vi "3D Axis Box Plot.vi"() -> ()   [LabVIEW 2022 SP3]
uses:
  <vilib>/Utility/miscctls.llb/LV3DPointTypeDef.ctl
  <vilib>/picture/3D Picture Control/Object/Create Object (drawable).vi
  <vilib>/picture/3D Picture Control/Object/Add Object (no reference).vi
  <vilib>/picture/3D Picture Control/NI_3D Picture Control.lvlib
panel:
  in  "Target":T1
  in  "Up Direction":T1
  in  "Camera Position":T1
  in  "Color 2":u32(colorbox)
  in  "Color":u32(colorbox)
  in  "Axis label?":bool
  in  "Half plane?":bool=TRUE
  in  "stop":bool
  out "3D Picture":refnum<vi>(3d-picture)
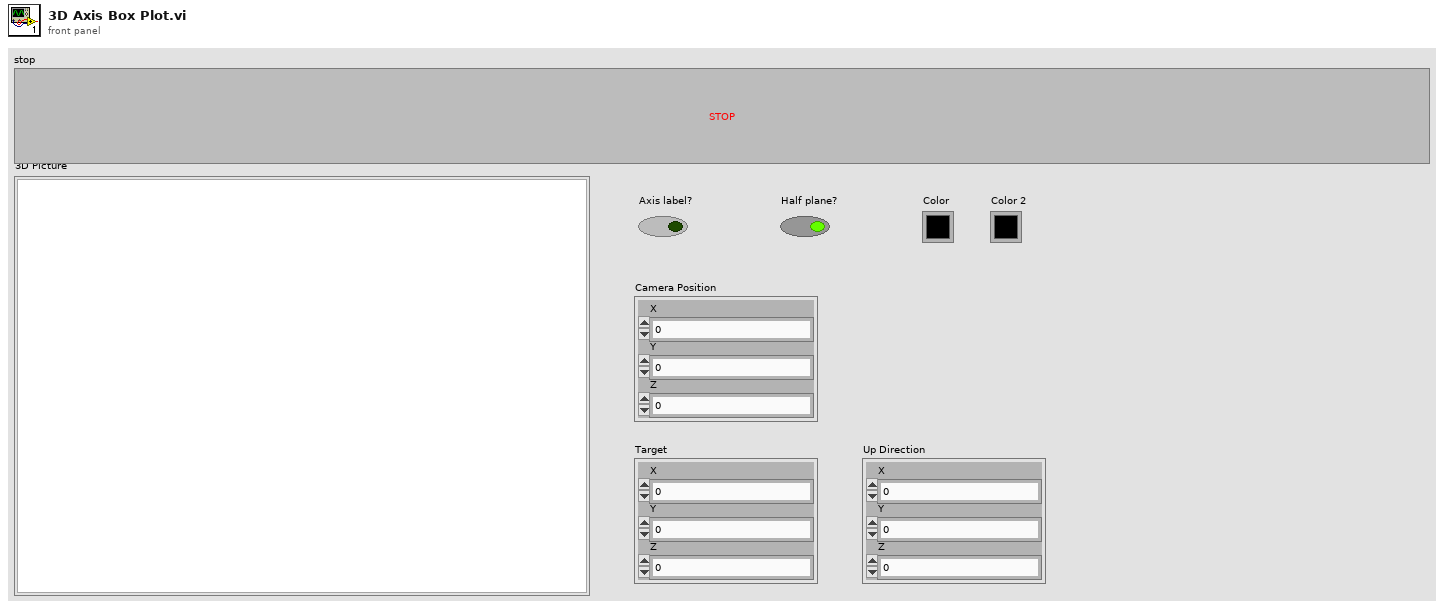
[diagram p1: front panel]
types:
  T1 = typedef "LV3DPointTypeDef.ctl" = cluster{"X":sgl, "Y":sgl, "Z":sgl}
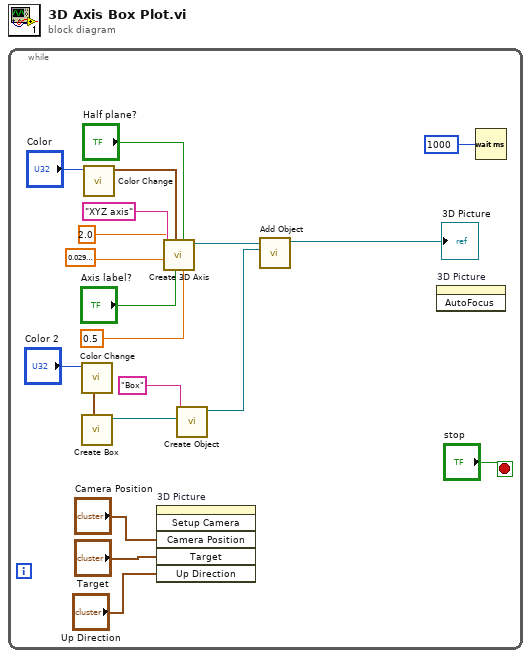
[diagram p0: block diagram]
diagram:
  n1 = while {
    stop <- "stop" stop-if-true
    n2 = call <vilib>:"Color Change.vi"("Color"="Color 2") -> ("RGBA"=w6:cluster{"R":sgl, "G":sgl, "B":sgl, "A":sgl})  [unwired: 10 in]
    n3 = call <vilib>:"Create Box.vi"("Color"=w6) -> ("New Box Refnum"=w18:refnum<vi>)  [unwired: 9 in, 1 out]
    n4 = call <vilib>:"Color Change.vi"("Color"="Color") -> ("RGBA"=w7:cluster{"R":sgl, "G":sgl, "B":sgl, "A":sgl})  [unwired: 10 in]
    n5 = invoke on="3D Picture" class="SceneGraphDisp (strict)" method="Setup Camera"("Camera Position"="Camera Position", "Target"="Target", "Up Direction"="Up Direction") -> ()  [unwired: 3 in, 6 out]
    n6 = call <vilib>:"Create 3D Axis.vi"("Character Size"=sgl 0.5, "Half plane?"="Half plane?", "Axis label?"="Axis label?", "Color"=w7, "Radius"=sgl 0.03, "Length"=sgl 2.0, "Name"="XYZ axis") -> ("New Object Refnum"=w17:refnum<vi>)  [unwired: 3 in, 1 out]
    n7 = call-poly <vilib>:"Create Object.vi"("Geometry"=w18, "Name"="Box") -> ("Scene:New Object"=w16:refnum<vi>)  [unwired: 8 in, 1 out]
    n8 = call-poly <vilib>:"Add Object.vi"("New Object In"=w16, "Scene Object In"=w17) -> ("Scene Object Out"=→"3D Picture":refnum<vi>)  [unwired: 8 in, 1 out]
    n9 = invoke on="3D Picture" class="SceneGraphDisp (strict)" method="AutoFocus"() -> ()  [unwired: 3 in, 3 out]
    n10 = Wait (ms)(milliseconds to wait=u32 1000 ("millisecond timer value")) -> ()  [unwired: 1 out]
  }
